vi "Graph.vi"() -> ()   [LabVIEW 2024]
uses:
  <vilib>/numeric/Random Number (Range) U64.vi
  <vilib>/numeric/sub_Random U32.vi
panel:
  out "Array":u64[](array[numeric])
  in  "Numeric":i32
  out "Waveform Chart":u64[](graph)
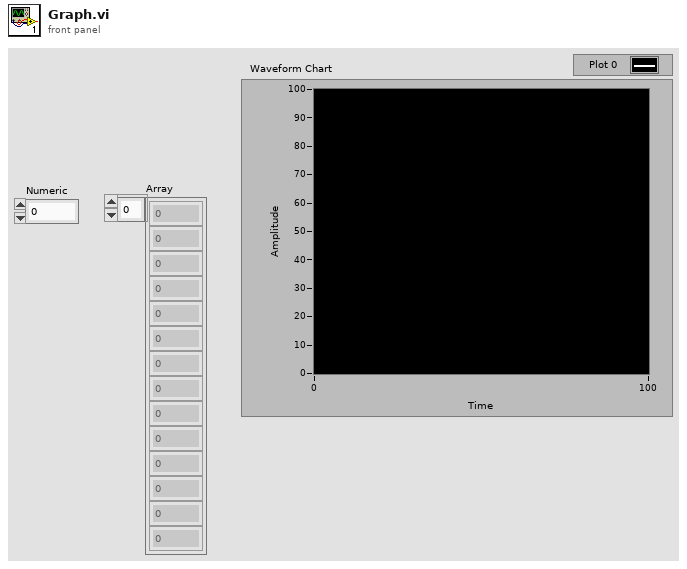
[diagram p1: front panel]
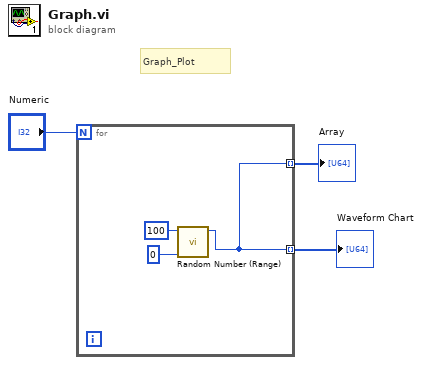
[diagram p0: block diagram]
diagram:
  # "Graph_Plot"
  n1 = for {
    N: "Numeric" -> [_]
    tunnel: [w4] -> w2 mode=indexing
    tunnel: [w4] -> w1 mode=indexing
    n2 = call-poly <vilib>:"Random Number (Range).vi"("lower bound (0)"=u64 0, "upper bound (100)"=u64 100) -> ("number"=w4:u64)  [unwired: 9 in]
  }
  "Waveform Chart" <- w2
  "Array" <- w1
